vi "Write Azimuth.vi"(8 "error in (no error)":errorcluster, 10 "Azimuth.lvclass":refnum<class "Azimuth.lvclass">, 11 "AzElParameters in":refnum<class "AzElParameters.lvclass">) -> (0 "error out":errorcluster, 3 "AzElParameters out":refnum<class "AzElParameters.lvclass">)   [LabVIEW 2014, in "TCSDataDefinitions.lvlib" / "TCSCommand.lvlib" / "TargetConfiguration.lvlib" / "Target.lvlib" / "FixedTarget.lvlib" / "AzElParameters.lvclass"]
uses:
  AzElParameters.lvclass
  Azimuth/Azimuth.lvclass
  AzElParameters.lvclass/AzElParameters.ctl
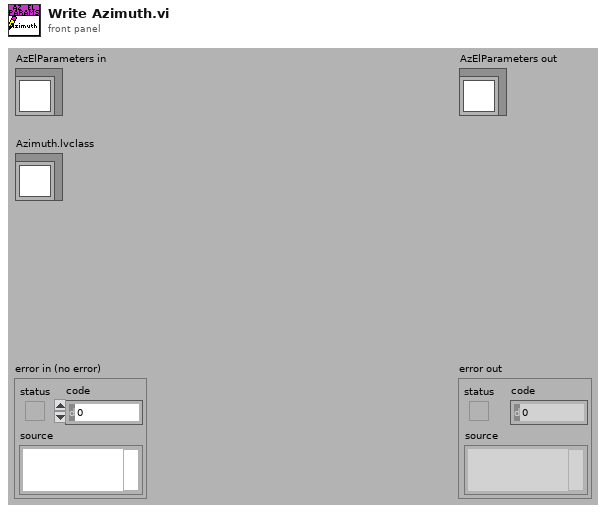
[diagram p1: front panel]
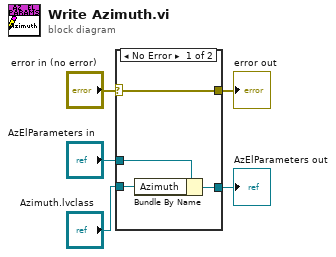
[diagram p0: block diagram]
diagram:
  n1 = case shown="No Error" "error in (no error)" {
    selector: "error in (no error)" -> [w9 w10]
    tunnel: [w9 w10] -> w4
    tunnel: [w7 w11] -> w2
    tunnel: "AzElParameters in" -> [w8 w11]
    tunnel: "Azimuth.lvclass" -> [w6 _]
    frame No Error {
      n2 = Bundle By Name(cluster=w8, "Azimuth"=w6) -> (w7:refnum<class "AzElParameters.lvclass">)
    }
    frame Error {
    }
  }
  "error out" <- w4
  "AzElParameters out" <- w2
